vi "wrapChildrenXML.vi"(7 "parentAttributeString":string, 8 "error in (no error)":errorcluster, 9 "childrenXML":string, 10 "parentName":string, 11 "WriteElement in":refnum<class "XMLGenerator.lvclass">) -> (0 "error out":errorcluster, 2 "XML out":string, 3 "WriteElement out":refnum<class "XMLGenerator.lvclass">)   [LabVIEW 2014, in "XML.lvlib" / "XMLGenerator.lvclass"]
doc: "This method adds all the XML elements together and formats them properly, including attributes, parent name and contents."
uses:
  <userlib>/Common/XML/XMLGenerator/XMLGenerator.lvclass
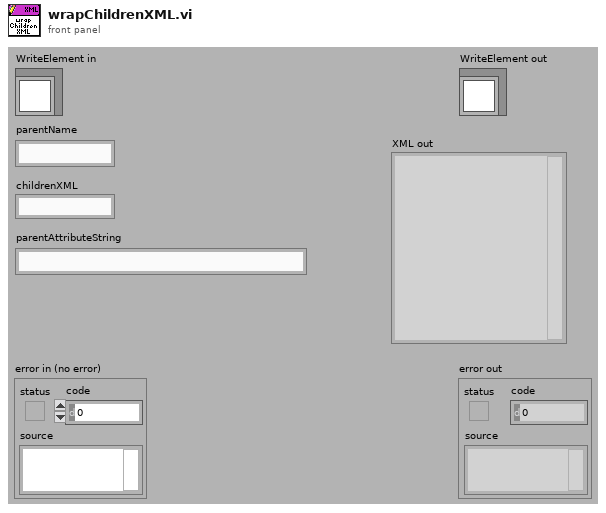
[diagram p1: front panel]
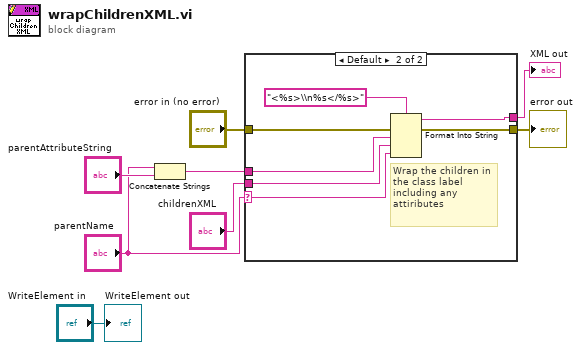
[diagram p0: block diagram]
diagram:
  n1 = Concatenate Strings("parentName", "parentAttributeString") -> (w3:string)
  n2 = case shown="Default" "parentName" {
    selector: "parentName" -> [_ w15]
    tunnel: [w9 w16] -> w2
    tunnel: "error in (no error)" -> [w10 w14]
    tunnel: [w10 w13] -> w6
    tunnel: w3 -> [_ w12]
    tunnel: "childrenXML" -> [w9 w11]
    frame "" {
      # "No class label,\nJust return children"
    }
    frame Default {
      # "Wrap the children in the class label\nincluding any attiributes"
      n3 = Format Into String(format string="<%s>\\n%s</%s>", error in=w14, w12, w11, w15) -> (resulting string=w16:string, error out=w13:errorcluster)  [unwired: 1 in]
    }
  }
  "error out" <- w6
  "XML out" <- w2
  "WriteElement out" <- "WriteElement in"
